vi "PI_SSH_CleanText.vi"(11 "Script":string) -> (3 "Array":string[](array[string]))   [LabVIEW 2019]
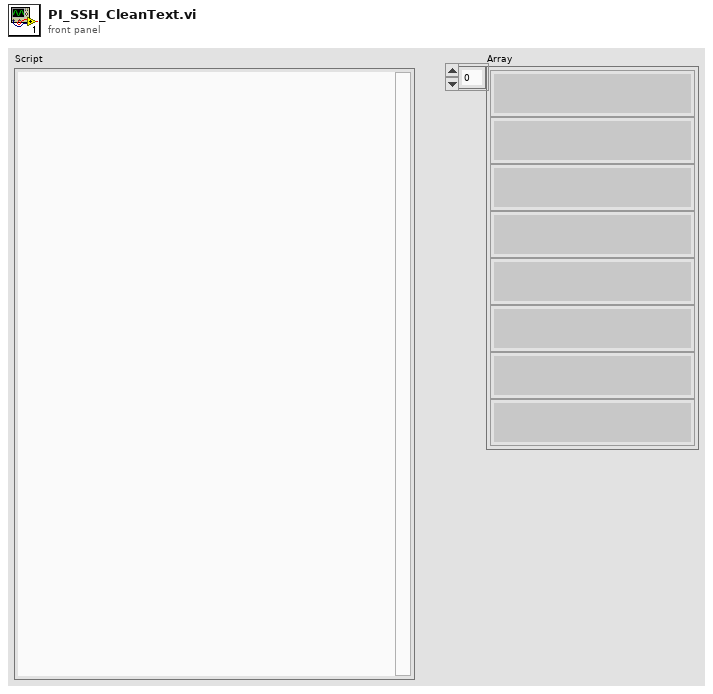
[diagram p1: front panel]
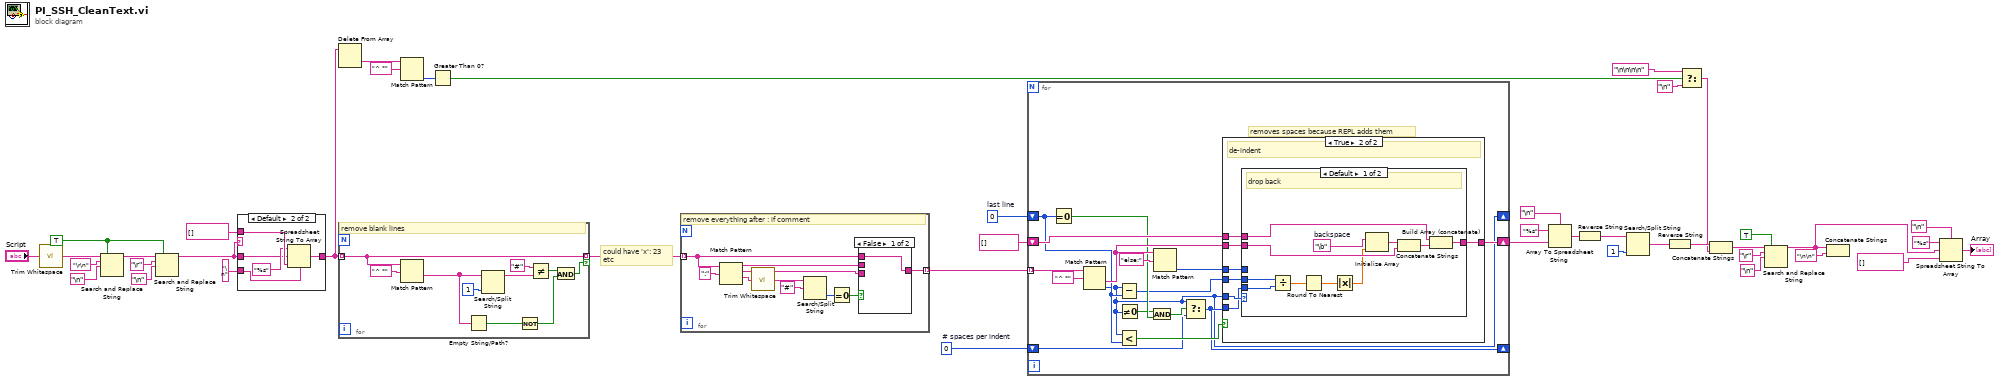
[diagram p0: block diagram]
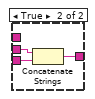
[diagram p3: hidden frame]
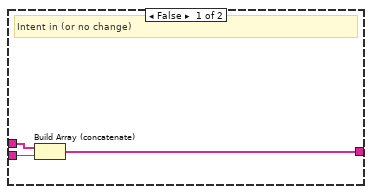
[diagram p4: hidden frame]
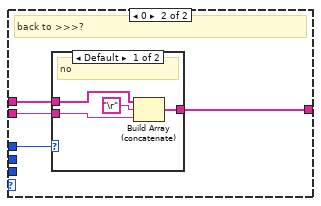
[diagram p5: hidden frame]
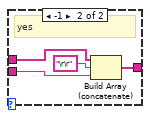
[diagram p6: hidden frame]
diagram:
  w8 = TRUE ("replace all? (F)")
  w32 = 0  # # spaces per indent
  w18 = 0  # last line
  # "could have 'x': 23\netc"
  n1 = call <vilib>:"Trim Whitespace.vi"("string"="Script") -> ("trimmed string"=w21:string)  [unwired: 1 in]
  n2 = Search and Replace String(replace all?=w8, input string=w21, search string="\r\n", replace string="\n" ("search string")) -> (result string=w7:string)  [unwired: 4 in, 3 out]
  n3 = Search and Replace String(replace all?=w8, input string=w7, search string="\r", replace string="\n" ("search string")) -> (result string=w9:string)  [unwired: 4 in, 3 out]
  n4 = case shown="Default" w9 {
    tunnel: string[] [] -> [w43 w48]
    tunnel: w9 -> [_ w45]
    tunnel: [w43 w44] -> w29
    tunnel: "\n" ("delimiter (LF)") -> [_ w47]
    frame "" {
    }
    frame Default {
      n5 = Spreadsheet String To Array(delimiter (Tab)=w47, format string="%s", spreadsheet string=w45, array type (2D Dbl)=w48) -> (array=w44:string[])
    }
  }
  n6 = Delete From Array(array=w29) -> (deleted portion=w14:string)  [unwired: 2 in, 1 out]
  n7 = for {
    tunnel: w29 -> [w57] mode=indexing
    tunnel: [w57] -> w30 mode=indexing if=w49
    # "remove blank lines"
    n8 = Match Pattern(string=w57, regular expression="^ *") -> (after substring=w54:string)  [unwired: 1 in, 3 out]
    n9 = Empty String/Path?(string/path=w54) -> (empty?=w56:bool)
    n10 = Search/Split String(string=w54, offset (0)=1) -> (substring before match=w53:string)  [unwired: 1 in, 2 out]
    n11 = Not(x=w56) -> (.not. x?=w50:bool)
    n12 = Not Equal?(x="#", y=w53) -> (x != y?=w51:bool)
    n13 = And(x=w51, y=w50) -> (x .and. y?=w49:bool)
  }
  n14 = Match Pattern(string=w14, regular expression="^ *") -> (offset past match=w12:i32)  [unwired: 1 in, 3 out]
  n15 = Greater Than 0?(x=w12) -> (x > 0?=w13:bool)
  n16 = for {
    tunnel: w30 -> [w65] mode=indexing
    tunnel: [w66] -> w31 mode=indexing
    # "remove everything after : if comment"
    n17 = Match Pattern(string=w65, regular expression=":") -> (before substring=w64:string, match substring=w67:string, after substring=w63:string)  [unwired: 1 in, 1 out]
    n18 = call <vilib>:"Trim Whitespace.vi"("string"=w63) -> ("trimmed string"=w62:string)  [unwired: 1 in]
    n19 = Search/Split String(string=w62, search string/char (-)="#") -> (offset of match=w60:i32)  [unwired: 1 in, 2 out]
    n20 = Equal To 0?(x=w60) -> (x = 0?=w59:bool)
    n21 = case shown="False" w59 {
      tunnel: w64 -> [_ w72]
      tunnel: w67 -> [_ w71]
      tunnel: [w69 w70] -> w66
      tunnel: w65 -> [w69 _]
      frame False {
      }
      frame True {
        n22 = Concatenate Strings(w72, w71) -> (w70:string)
      }
    }
  }
  n23 = for {
    tunnel: w31 -> [w85] mode=indexing
    shift-right: [w73] -> _
    shift-left: w18 -> [w76]
    shift-right: [w84] -> w20
    shift-left: string[] [] ("Array") -> [w86]
    shift-right: [w74] -> _
    shift-left: w32 -> [w77]
    # "removes spaces because REPL adds them"
    n24 = Equal To 0?(x=w76) -> (x = 0?=w80:bool)
    n25 = Match Pattern(string=w85, regular expression="^ *") -> (after substring=w83:string, offset past match=w73:i32)  [unwired: 1 in, 2 out]
    n26 = Subtract(x=w73, y=w76) -> (x-y=w75:i32)
    n27 = Less?(x=w73, y=w76) -> (x < y?=w87:bool)
    n28 = Not Equal To 0?(x=w73) -> (x != 0?=w79:bool)
    n29 = And(x=w79, y=w80) -> (x .and. y?=w78:bool)
    n30 = Match Pattern(string=w83, regular expression="else:") -> (offset past match=w81:i32)  [unwired: 1 in, 3 out]
    n31 = Select(t=w73, s=w78, f=w77) -> (s? t:f=w74:i32)
    n32 = case shown="True" w87 {
      tunnel: w86 -> [w91 w98]
      tunnel: w83 -> [w90 w96]
      tunnel: [w89 w97] -> w84
      tunnel: w73 -> [_ w95]
      tunnel: w81 -> [_ w94]
      tunnel: w75 -> [_ w93]
      tunnel: w74 -> [_ w92]
      frame False {
        # "Intent in (or no change)"
        n33 = Build Array (concatenate)(w91, w90) -> (w89:string[])
      }
      frame True {
        # "de-indent"
        n34 = case shown="Default" w95 {
          tunnel: w98 -> [w109 w113]
          tunnel: [w108 w112] -> w97
          tunnel: w96 -> [w107 w111]
          tunnel: w94 -> [_ w110]
          tunnel: w93 -> [w102 _]
          tunnel: w92 -> [w101 _]
          frame Default {
            w105 = "\b"  # backspace
            # "drop back"
            n35 = Divide(x=w102, y=w101) -> (x/y=w100:dbl)
            n36 = Round To Nearest(number=w100) -> (nearest integer value=w99:dbl)
            n37 = Absolute Value(x=w99) -> (abs(x)=w103:dbl)
            n38 = Initialize Array(w105, w103) -> (w104:string[])
            n39 = Concatenate Strings(w104, w107) -> (w106:string)
            n40 = Build Array (concatenate)(w109, w106) -> (w108:string[])
          }
          frame 0 {
            # "back to >>>?"
            n41 = case shown="Default" w110 {
              tunnel: w113 -> [w116 w121]
              tunnel: [w115 w120] -> w112
              tunnel: w111 -> [w114 w119]
              frame Default {
                # "no"
                n42 = Build Array (concatenate)(w116, "\r" ("regular expression"), w114) -> (w115:string[])
              }
              frame -1 {
                # "yes"
                n43 = Build Array (concatenate)(w121, "\r\r" ("regular expression"), w119) -> (w120:string[])
              }
            }
          }
        }
      }
    }
  }
  n44 = Array To Spreadsheet String(delimiter (Tab)="\n", array=w20, 3:"%s" ("format string")) -> (spreadsheet string=w24:string)
  n45 = Reverse String(1:w24) -> (0:w25:string)
  n46 = Search/Split String(string=w25, offset (0)=1) -> (match + rest of string=w27:string)  [unwired: 1 in, 2 out]
  n47 = Reverse String(1:w27) -> (0:w28:string)
  n48 = Select(t="\n\n\n\n", s=w13, f="\n") -> (s? t:f=w17:string)
  n49 = Concatenate Strings(w28, w17) -> (w38:string)
  n50 = Search and Replace String(replace all?=TRUE ("replace all? (F)"), input string=w38, search string="\r", replace string="\n" ("replace string (\"\")")) -> (result string=w1:string)  [unwired: 4 in, 3 out]
  n51 = Concatenate Strings(w1, "\n\n" ("string")) -> ()  [unwired: 1 out]
  n52 = Spreadsheet String To Array(delimiter (Tab)="\n", format string="%s", spreadsheet string=w1, array type (2D Dbl)=string[] []) -> (array=→"Array":string[])
